vi "nanocal -- nuclear schottky fit V7.vi"() -> ()   [LabVIEW 2021] (continued)
  out "string OUT":string="  \"IDS0158_210310_RAW_cal__ref_\" ->   <|    \"ζ\" -> 0.338724462580   ,  \"τ1\" -> 0.031757745266   ,  \"τS\" -> 0.247286819047   ,  \"τN\" -> 0.322740818116   ,  \"τC\" -> 0.001034291318   ,  \"κ0\" -> 0.000000000505   ,  \"mm1\" -> 0.000261080239   ,  \"mm2\" -> 0.013473055910   ,  \"mm3\" -> 0.782167842652   ,  \"T\" -> 0.140000000000   ,  \"B\" -> 12.000000000000   ,  \"θ\" -> 0.000000000000   ,  \"Reoff\" -> -114641566.265060246000   ,  \"Imoff\" -> 0.000000000000   ,  \"στ1\" -> 0.023975320210   ,  \"στS\" -> 0.076414054009   ,  \"στN\" -> 0.076454917520    |>   , \r\"IDS0158_210310_RAW_cal__sam_\" ->   <|    \"ζ\" -> 0.286336668596   ,  \"τ1\" -> 0.037477267671   ,  \"τS\" -> 0.354459287884   ,  \"τN\" -> 0.444916383639   ,  \"τC\" -> 0.001225600579   ,  \"κ0\" -> 0.000000000596   ,  \"mm1\" -> 0.000272242393   ,  \"mm2\" -> 0.016302418461   ,  \"mm3\" -> 1.050394445660   ,  \"T\" -> 0.140000000000   ,  \"B\" -> 12.000000000000   ,  \"θ\" -> 0.000000000000   ,  \"Reoff\" -> 0.000000000000   ,  \"Imoff\" -> 0.000000000000   ,  \"στ1\" -> 0.000000000000   ,  \"στS\" -> 0.000000000000   ,  \"στN\" -> 0.000000000000    |>   , \r\"IDS0159_210310_RAW_cal__ref_\" ->   <|    \"ζ\" -> 0.271267920492   ,  \"τ1\" -> 0.029985631647   ,  \"τS\" -> 0.193691005295   ,  \"τN\" -> 0.182171075098   ,  \"τC\" -> 0.001008816819   ,  \"κ0\" -> 0.000000000648   ,  \"mm1\" -> 0.000214568285   ,  \"mm2\" -> 0.015007137955   ,  \"mm3\" -> 0.493594147559   ,  \"T\" -> 0.170000000000   ,  \"B\" -> 12.000000000000   ,  \"θ\" -> 0.000000000000   ,  \"Reoff\" -> -68518072.289156615700   ,  \"Imoff\" -> 0.000000000000   ,  \"στ1\" -> 0.012908928279   ,  \"στS\" -> 0.012278249433   ,  \"στN\" -> 0.000000000000    |>   , \r\"IDS0159_210310_RAW_cal__sam_\" ->   <|    \"ζ\" -> 0.219100303741   ,  \"τ1\" -> 0.028643012604   ,  \"τS\" -> 0.279362928811   ,  \"τN\" -> 0.246156444058   ,  \"τC\" -> 0.001272401549   ,  \"κ0\" -> 0.000000000760   ,  \"mm1\" -> 0.000227975653   ,  \"mm2\" -> 0.014929571562   ,  \"mm3\" -> 0.655418694024   ,  \"T\" -> 0.170000000000   ,  \"B\" -> 12.000000000000   ,  \"θ\" -> 0.000000000000   ,  \"Reoff\" -> 0.000000000000   ,  \"Imoff\" -> 0.000000000000   ,  \"στ1\" -> 0.000000000000   ,  \"στS\" -> 0.000000000000   ,  \"στN\" -> 0.000000000000    |>   , \r\"IDS0160_210310_RAW_cal__ref_\" ->   <|    \"ζ\" -> 0.207139977904   ,  \"τ1\" -> 0.027467343957   ,  \"τS\" -> 0.117438673826   ,  \"τN\" -> 0.102057074143   ,  \"τC\" -> 0.000949663971   ,  \"κ0\" -> 0.000000000917   ,  \"mm1\" -> 0.000162053218   ,  \"mm2\" -> 0.014024936030   ,  \"mm3\" -> 0.279192111033   ,  \"T\" -> 0.200000000000   ,  \"B\" -> 12.000000000000   ,  \"θ\" -> 0.000000000000   ,  \"Reoff\" -> -40668674.698795177000   ,  \"Imoff\" -> 0.000000000000   ,  \"στ1\" -> 0.009618369087   ,  \"στS\" -> 0.007137384425   ,  \"στN\" -> 0.000000000000    |>   , \r\"IDS0160_210310_RAW_cal__sam_\" ->   <|    \"ζ\" -> 0.170488637524   ,  \"τ1\" -> 0.029234231120   ,  \"τS\" -> 0.149095458227   ,  \"τN\" -> 0.151792620275   ,  \"τC\" -> 0.001113424175   ,  \"κ0\" -> 0.000000001042   ,  \"mm1\" -> 0.000161291869   ,  \"mm2\" -> 0.013922632736   ,  \"mm3\" -> 0.368449807743   ,  \"T\" -> 0.200000000000   ,  \"B\" -> 12.000000000000   ,  \"θ\" -> 0.000000000000   ,  \"Reoff\" -> 0.000000000000   ,  \"Imoff\" -> 0.000000000000   ,  \"στ1\" -> 0.000000000000   ,  \"στS\" -> 0.000000000000   ,  \"στN\" -> 0.000000000000    |>   , \r\"IDS0161_210310_RAW_cal__ref_\" ->   <|    \"ζ\" -> 0.165651103495   ,  \"τ1\" -> 0.025219369633   ,  \"τS\" -> 0.095243887499   ,  \"τN\" -> 0.068405844588   ,  \"τC\" -> 0.001096621932   ,  \"κ0\" -> 0.000000001058   ,  \"mm1\" -> 0.000154524257   ,  \"mm2\" -> 0.013909362731   ,  \"mm3\" -> 0.203010595371   ,  \"T\" -> 0.220000000000   ,  \"B\" -> 12.000000000000   ,  \"θ\" -> 0.000000000000   ,  \"Reoff\" -> -26138554.216867461800   ,  \"Imoff\" -> 0.000000000000   ,  \"στ1\" -> 0.007587881902   ,  \"στS\" -> 0.004844828321   ,  \"στN\" -> 0.000000000000    |>   , \r\"IDS0161_210310_RAW_cal__sam_\" ->   <|    \"ζ\" -> 0.130531197151   ,  \"τ1\" -> 0.025704482770   ,  \"τS\" -> 0.129606657196   ,  \"τN\" -> 0.091602369165   ,  \"τC\" -> 0.001441379995   ,  \"κ0\" -> 0.000000001211   ,  \"mm1\" -> 0.000164978070   ,  \"mm2\" -> 0.014468182937   ,  \"mm3\" -> 0.262596407151   ,  \"T\" -> 0.220000000000   ,  \"B\" -> 12.000000000000   ,  \"θ\" -> 0.000000000000   ,  \"Reoff\" -> 0.000000000000   ,  \"Imoff\" -> 0.000000000000   ,  \"στ1\" -> 0.000000000000   ,  \"στS\" -> 0.000000000000   ,  \"στN\" -> 0.000000000000    |>   , \r\"IDS0162_210310_RAW_cal__ref_\" ->   <|    \"ζ\" -> 0.096222034275   ,  \"τ1\" -> 0.023686784650   ,  \"τS\" -> 0.070336744639   ,  \"τN\" -> 0.023939989572   ,  \"τC\" -> 0.001388596335   ,  \"κ0\" -> 0.000000001367   ,  \"mm1\" -> 0.000119909077   ,  \"mm2\" -> 0.016622969082   ,  \"mm3\" -> 0.111680736187   ,  \"T\" -> 0.280000000000   ,  \"B\" -> 12.000000000000   ,  \"θ\" -> 0.000000000000   ,  \"Reoff\" -> -11003012.048192769300   ,  \"Imoff\" -> 0.000000000000   ,  \"στ1\" -> 0.008753356754   ,  \"στS\" -> 0.002669913437   ,  \"στN\" -> 0.000000000000    |>   , \r\"IDS0162_210310_RAW_cal__sam_\" ->   <|    \"ζ\" -> 0.078258046754   ,  \"τ1\" -> 0.028009840731   ,  \"τS\" -> 0.092122038762   ,  \"τN\" -> 0.030129595899   ,  \"τC\" -> 0.001641062244   ,  \"κ0\" -> 0.000000001543   ,  \"mm1\" -> 0.000117303440   ,  \"mm2\" -> 0.019983073008   ,  \"mm3\" -> 0.141369335330   ,  \"T\" -> 0.280000000000   ,  \"B\" -> 12.000000000000   ,  \"θ\" -> 0.000000000000   ,  \"Reoff\" -> 0.000000000000   ,  \"Imoff\" -> 0.000000000000   ,  \"στ1\" -> 0.000000000000   ,  \"στS\" -> 0.000000000000   ,  \"στN\" -> 0.000000000000    |>   , \r\"IDS0163_210310_RAW_cal__ref_\" ->   <|    \"ζ\" -> 0.066672200447   ,  \"τ1\" -> 0.021639337174   ,  \"τS\" -> 0.054330230678   ,  \"τN\" -> 0.012190158529   ,  \"τC\" -> 0.001673698086   ,  \"κ0\" -> 0.000000001744   ,  \"mm1\" -> 0.000101848885   ,  \"mm2\" -> 0.016608176692   ,  \"mm3\" -> 0.077558459612   ,  \"T\" -> 0.330000000000   ,  \"B\" -> 12.000000000000   ,  \"θ\" -> 0.000000000000   ,  \"Reoff\" -> -6192771.084337353710   ,  \"Imoff\" -> 0.000000000000   ,  \"στ1\" -> 0.010795838687   ,  \"στS\" -> 0.002003612837   ,  \"στN\" -> 0.000000000000    |>   , \r\"IDS0163_210310_RAW_cal__sam_\" ->   <|    \"ζ\" -> 0.054088186012   ,  \"τ1\" -> 0.023838802615   ,  \"τS\" -> 0.069079396629   ,  \"τN\" -> 0.016435267456   ,  \"τC\" -> 0.002025071743   ,  \"κ0\" -> 0.000000001955   ,  \"mm1\" -> 0.000101234646   ,  \"mm2\" -> 0.018244822177   ,  \"mm3\" -> 0.097657814678   ,  \"T\" -> 0.330000000000   ,  \"B\" -> 12.000000000000   ,  \"θ\" -> 0.000000000000   ,  \"Reoff\" -> 0.000000000000   ,  \"Imoff\" -> 0.000000000000   ,  \"στ1\" -> 0.000000000000   ,  \"στS\" -> 0.000000000000   ,  \"στN\" -> 0.000000000000    |>   , \r\"IDS0164_210310_RAW_cal__ref_\" ->   <|    \"ζ\" -> 0.047185670549   ,  \"τ1\" -> 0.020999787986   ,  \"τS\" -> 0.044123234525   ,  \"τN\" -> 0.006414229914   ,  \"τC\" -> 0.002330922094   ,  \"κ0\" -> 0.000000002161   ,  \"mm1\" -> 0.000100189786   ,  \"mm2\" -> 0.017276594586   ,  \"mm3\" -> 0.058876034294   ,  \"T\" -> 0.400000000000   ,  \"B\" -> 12.000000000000   ,  \"θ\" -> 0.000000000000   ,  \"Reoff\" -> -3126506.024096369740   ,  \"Imoff\" -> 0.000000000000   ,  \"στ1\" -> 0.014319461595   ,  \"στS\" -> 0.001588428387   ,  \"στN\" -> 0.000000000000    |>   , \r\"IDS0164_210310_RAW_cal__sam_\" ->   <|    \"ζ\" -> 0.039314966212   ,  \"τ1\" -> 0.020712803909   ,  \"τS\" -> 0.055413767550   ,  \"τN\" -> 0.008474403424   ,  \"τC\" -> 0.002674063387   ,  \"κ0\" -> 0.000000002415   ,  \"mm1\" -> 0.000096818147   ,  \"mm2\" -> 0.017190811405   ,  \"mm3\" -> 0.072499170001   ,  \"T\" -> 0.400000000000   ,  \"B\" -> 12.000000000000   ,  \"θ\" -> 0.000000000000   ,  \"Reoff\" -> 0.000000000000   ,  \"Imoff\" -> 0.000000000000   ,  \"στ1\" -> 0.000000000000   ,  \"στS\" -> 0.000000000000   ,  \"στN\" -> 0.000000000000    |>   , \r\"IDS0165_210310_RAW_cal__ref_\" ->   <|    \"ζ\" -> 0.033577393126   ,  \"τ1\" -> 0.018946820322   ,  \"τS\" -> 0.035749921348   ,  \"τN\" -> 0.004008447047   ,  \"τC\" -> 0.003122429757   ,  \"κ0\" -> 0.000000002680   ,  \"mm1\" -> 0.000093748549   ,  \"mm2\" -> 0.016142439680   ,  \"mm3\" -> 0.046926412611   ,  \"T\" -> 0.480000000000   ,  \"B\" -> 12.000000000000   ,  \"θ\" -> 0.000000000000   ,  \"Reoff\" -> -1313253.012048184870   ,  \"Imoff\" -> 0.000000000000   ,  \"στ1\" -> 0.017565086331   ,  \"στS\" -> 0.001375721175   ,  \"στN\" -> 0.000000000000    |>   , \r\"IDS0165_210310_RAW_cal__sam_\" ->   <|    \"ζ\" -> 0.031945976845   ,  \"τ1\" -> 0.019000922826   ,  \"τS\" -> 0.045624146388   ,  \"τN\" -> 0.005314716063   ,  \"τC\" -> 0.002488383471   ,  \"κ0\" -> 0.000000002954   ,  \"mm1\" -> 0.000073272643   ,  \"mm2\" -> 0.016306894362   ,  \"mm3\" -> 0.057675293464   ,  \"T\" -> 0.480000000000   ,  \"B\" -> 12.000000000000   ,  \"θ\" -> 0.000000000000   ,  \"Reoff\" -> 0.000000000000   ,  \"Imoff\" -> 0.000000000000   ,  \"στ1\" -> 0.000000000000   ,  \"στS\" -> 0.000000000000   ,  \"στN\" -> 0.000000000000    |>   , \r\"IDS0166_210310_RAW_cal__ref_\" ->   <|    \"ζ\" -> 0.026134408941   ,  \"τ1\" -> 0.018837221506   ,  \"τS\" -> 0.029046436266   ,  \"τN\" -> 0.002475934064   ,  \"τC\" -> 0.003637611641   ,  \"κ0\" -> 0.000000003369   ,  \"mm1\" -> 0.000082770074   ,  \"mm2\" -> 0.016386102123   ,  \"mm3\" -> 0.038352149797   ,  \"T\" -> 0.580000000000   ,  \"B\" -> 12.000000000000   ,  \"θ\" -> 0.000000000000   ,  \"Reoff\" -> -406626.506024092435   ,  \"Imoff\" -> 0.000000000000   ,  \"στ1\" -> 0.034768871814   ,  \"στS\" -> 0.001627850434   ,  \"στN\" -> 0.000000000000    |>   , \r\"IDS0166_210310_RAW_cal__sam_\" ->   <|    \"ζ\" -> 0.023031239946   ,  \"τ1\" -> 0.018268814012   ,  \"τS\" -> 0.037269400776   ,  \"τN\" -> 0.002696792890   ,  \"τC\" -> 0.003257395394   ,  \"κ0\" -> 0.000000003720   ,  \"mm1\" -> 0.000067670174   ,  \"mm2\" -> 0.016445281937   ,  \"mm3\" -> 0.045899921957   ,  \"T\" -> 0.580000000000   ,  \"B\" -> 12.000000000000   ,  \"θ\" -> 0.000000000000   ,  \"Reoff\" -> 0.000000000000   ,  \"Imoff\" -> 0.000000000000   ,  \"στ1\" -> 0.000000000000   ,  \"στS\" -> 0.000000000000   ,  \"στN\" -> 0.000000000000    |>   , \r\"IDS0167_210310_RAW_cal__ref_\" ->   <|    \"ζ\" -> 0.026557278794   ,  \"τ1\" -> 0.016933945977   ,  \"τS\" -> 0.022881111855   ,  \"τN\" -> 0.001392473895   ,  \"τC\" -> 0.004119437148   ,  \"κ0\" -> 0.000000003981   ,  \"mm1\" -> 0.000090964667   ,  \"mm2\" -> 0.015177563241   ,  \"mm3\" -> 0.030703081351   ,  \"T\" -> 0.680000000000   ,  \"B\" -> 12.000000000000   ,  \"θ\" -> 0.000000000000   ,  \"Reoff\" -> 0.000000000000   ,  \"Imoff\" -> 0.000000000000   ,  \"στ1\" -> 0.000000000000   ,  \"στS\" -> 0.000000000000   ,  \"στN\" -> 0.000000000000    |>   , \r\"IDS0167_210310_RAW_cal__sam_\" ->   <|    \"ζ\" -> 0.019920170845   ,  \"τ1\" -> 0.016368892412   ,  \"τS\" -> 0.030579536580   ,  \"τN\" -> 0.001736017565   ,  \"τC\" -> 0.004971418152   ,  \"κ0\" -> 0.000000004410   ,  \"mm1\" -> 0.000083939556   ,  \"mm2\" -> 0.015095997595   ,  \"mm3\" -> 0.039119658918   ,  \"T\" -> 0.680000000000   ,  \"B\" -> 12.000000000000   ,  \"θ\" -> 0.000000000000   ,  \"Reoff\" -> 0.000000000000   ,  \"Imoff\" -> 0.000000000000   ,  \"στ1\" -> 0.000000000000   ,  \"στS\" -> 0.000000000000   ,  \"στN\" -> 0.000000000000    |>   , \r\"IDS0168_210310_RAW_cal__ref_\" ->   <|    \"ζ\" -> 0.022041296958   ,  \"τ1\" -> 0.014045615335   ,  \"τS\" -> 0.018889590451   ,  \"τN\" -> 0.000813465770   ,  \"τC\" -> 0.004122617309   ,  \"κ0\" -> 0.000000005540   ,  \"mm1\" -> 0.000073491061   ,  \"mm2\" -> 0.013002629707   ,  \"mm3\" -> 0.025229449010   ,  \"T\" -> 0.910000000000   ,  \"B\" -> 12.000000000000   ,  \"θ\" -> 0.000000000000   ,  \"Reoff\" -> 0.000000000000   ,  \"Imoff\" -> 0.000000000000   ,  \"στ1\" -> 0.000000000000   ,  \"στS\" -> 0.000000000000   ,  \"στN\" -> 0.000000000000    |>   , \r\"IDS0168_210310_RAW_cal__sam_\" ->   <|    \"ζ\" -> 0.017558473054   ,  \"τ1\" -> 0.014545104284   ,  \"τS\" -> 0.022979681288   ,  \"τN\" -> 0.000840829385   ,  \"τC\" -> 0.005228030240   ,  \"κ0\" -> 0.000000006068   ,  \"mm1\" -> 0.000073916527   ,  \"mm2\" -> 0.013750428362   ,  \"mm3\" -> 0.030187552103   ,  \"T\" -> 0.910000000000   ,  \"B\" -> 12.000000000000   ,  \"θ\" -> 0.000000000000   ,  \"Reoff\" -> 0.000000000000   ,  \"Imoff\" -> 0.000000000000   ,  \"στ1\" -> 0.000000000000   ,  \"στS\" -> 0.000000000000   ,  \"στN\" -> 0.000000000000    |>   , \r\"IDS0169_210310_RAW_cal__ref_\" ->   <|    \"ζ\" -> 0.021090283514   ,  \"τ1\" -> 0.013945744068   ,  \"τS\" -> 0.014386606899   ,  \"τN\" -> 0.000345175874   ,  \"τC\" -> 0.004902956629   ,  \"κ0\" -> 0.000000007742   ,  \"mm1\" -> 0.000076221408   ,  \"mm2\" -> 0.013209066715   ,  \"mm3\" -> 0.020605892822   ,  \"T\" -> 1.230000000000   ,  \"B\" -> 12.000000000000   ,  \"θ\" -> 0.000000000000   ,  \"Reoff\" -> 0.000000000000   ,  \"Imoff\" -> 0.000000000000   ,  \"στ1\" -> 0.000000000000   ,  \"στS\" -> 0.000000000000   ,  \"στN\" -> 0.000000000000    |>   , \r\"IDS0169_210310_RAW_cal__sam_\" ->   <|    \"ζ\" -> 0.011916480594   ,  \"τ1\" -> 0.012551282481   ,  \"τS\" -> 0.018233218660   ,  \"τN\" -> 0.000345702746   ,  \"τC\" -> 0.004699451527   ,  \"κ0\" -> 0.000000008451   ,  \"mm1\" -> 0.000044190864   ,  \"mm2\" -> 0.012162820727   ,  \"mm3\" -> 0.023844039179   ,  \"T\" -> 1.230000000000   ,  \"B\" -> 12.000000000000   ,  \"θ\" -> 0.000000000000   ,  \"Reoff\" -> 0.000000000000   ,  \"Imoff\" -> 0.000000000000   ,  \"στ1\" -> 0.000000000000   ,  \"στS\" -> 0.000000000000   ,  \"στN\" -> 0.000000000000    |>   , \r\"IDS0170_210310_RAW_cal__ref_\" ->   <|    \"ζ\" -> 0.021449250230   ,  \"τ1\" -> 0.014564522147   ,  \"τS\" -> 0.008878867204   ,  \"τN\" -> 0.000064984242   ,  \"τC\" -> 0.006207353748   ,  \"κ0\" -> 0.000000012530   ,  \"mm1\" -> 0.000077778127   ,  \"mm2\" -> 0.013872772336   ,  \"mm3\" -> 0.015957015786   ,  \"T\" -> 1.970000000000   ,  \"B\" -> 12.000000000000   ,  \"θ\" -> 0.000000000000   ,  \"Reoff\" -> 0.000000000000   ,  \"Imoff\" -> 0.000000000000   ,  \"στ1\" -> 0.000000000000   ,  \"στS\" -> 0.000000000000   ,  \"στN\" -> 0.000000000000    |>   , \r\"IDS0170_210310_RAW_cal__sam_\" ->   <|    \"ζ\" -> 0.012831327568   ,  \"τ1\" -> 0.013315909415   ,  \"τS\" -> 0.012590836847   ,  \"τN\" -> 0.000065003013   ,  \"τC\" -> 0.005276356243   ,  \"κ0\" -> 0.000000013610   ,  \"mm1\" -> 0.000047406274   ,  \"mm2\" -> 0.013137605540   ,  \"mm3\" -> 0.018225484932   ,  \"T\" -> 1.970000000000   ,  \"B\" -> 12.000000000000   ,  \"θ\" -> 0.000000000000   ,  \"Reoff\" -> 0.000000000000   ,  \"Imoff\" -> 0.000000000000   ,  \"στ1\" -> 0.000000000000   ,  \"στS\" -> 0.000000000000   ,  \"στN\" -> 0.000000000000    |>   , \r\"IDS0171_210310_RAW_cal__ref_\" ->   <|    \"ζ\" -> 0.024633693577   ,  \"τ1\" -> 0.014940694735   ,  \"τS\" -> 0.006137734482   ,  \"τN\" -> 0.000014567254   ,  \"τC\" -> 0.005080683927   ,  \"κ0\" -> 0.000000022488   ,  \"mm1\" -> 0.000067969819   ,  \"mm2\" -> 0.011256263587   ,  \"mm3\" -> 0.015001000908   ,  \"T\" -> 3.190000000000   ,  \"B\" -> 12.000000000000   ,  \"θ\" -> 0.000000000000   ,  \"Reoff\" -> 0.000000000000   ,  \"Imoff\" -> 0.000000000000   ,  \"στ1\" -> 0.000000000000   ,  \"στS\" -> 0.000000000000   ,  \"στN\" -> 0.000000000000    |>   , \r\"IDS0171_210310_RAW_cal__sam_\" ->   <|    \"ζ\" -> 0.019774146838   ,  \"τ1\" -> 0.013257273421   ,  \"τS\" -> 0.007064131508   ,  \"τN\" -> 0.000028000819   ,  \"τC\" -> 0.006942241845   ,  \"κ0\" -> 0.000000023477   ,  \"mm1\" -> 0.000068886863   ,  \"mm2\" -> 0.012935419574   ,  \"mm3\" -> 0.014427582022   ,  \"T\" -> 3.190000000000   ,  \"B\" -> 12.000000000000   ,  \"θ\" -> 0.000000000000   ,  \"Reoff\" -> 0.000000000000   ,  \"Imoff\" -> 0.000000000000   ,  \"στ1\" -> 0.000000000000   ,  \"στS\" -> 0.000000000000   ,  \"στN\" -> 0.000000000000    |>   , \r\"IDS0172_210310_RAW_cal__ref_\" ->   <|    \"ζ\" -> 0.027835388666   ,  \"τ1\" -> 0.013976390421   ,  \"τS\" -> 0.003539188638   ,  \"τN\" -> 0.000003774856   ,  \"τC\" -> 0.004420299329   ,  \"κ0\" -> 0.000000055482   ,  \"mm1\" -> 0.000054408485   ,  \"mm2\" -> 0.007998445403   ,  \"mm3\" -> 0.013985419121   ,  \"T\" -> 5.800000000000   ,  \"B\" -> 12.000000000000   ,  \"θ\" -> 0.000000000000   ,  \"Reoff\" -> 0.000000000000   ,  \"Imoff\" -> 0.000000000000   ,  \"στ1\" -> 0.000000000000   ,  \"στS\" -> 0.000000000000   ,  \"στN\" -> 0.000000000000    |>   , \r\"IDS0172_210310_RAW_cal__sam_\" ->   <|    \"ζ\" -> 0.029251354442   ,  \"τ1\" -> 0.014634751206   ,  \"τS\" -> 0.003873958746   ,  \"τN\" -> 0.000007000487   ,  \"τC\" -> 0.006827504775   ,  \"κ0\" -> 0.000000056438   ,  \"mm1\" -> 0.000072018576   ,  \"mm2\" -> 0.010723236476   ,  \"mm3\" -> 0.014661483476   ,  \"T\" -> 5.800000000000   ,  \"B\" -> 12.000000000000   ,  \"θ\" -> 0.000000000000   ,  \"Reoff\" -> 0.000000000000   ,  \"Imoff\" -> 0.000000000000   ,  \"στ1\" -> 0.000000000000   ,  \"στS\" -> 0.000000000000   ,  \"στN\" -> 0.000000000000    |>   , \r\"IDS0181_210310_RAW_cal__ref_\" ->   <|    \"ζ\" -> 0.196256884521   ,  \"τ1\" -> 0.071380539398   ,  \"τS\" -> 0.034448108903   ,  \"τN\" -> 0.119444210569   ,  \"τC\" -> 0.001245873609   ,  \"κ0\" -> 0.000000000908   ,  \"mm1\" -> 0.000199286041   ,  \"mm2\" -> 0.012356130491   ,  \"mm3\" -> 0.244165743118   ,  \"T\" -> 0.179000000000   ,  \"B\" -> 12.000000000000   ,  \"θ\" -> 90.000000000000   ,  \"Reoff\" -> -32111445.783132523300   ,  \"Imoff\" -> 0.000000000000   ,  \"στ1\" -> 0.005873597921   ,  \"στS\" -> 0.002285203630   ,  \"στN\" -> 0.000000000000    |>   , \r\"IDS0181_210310_RAW_cal__sam_\" ->   <|    \"ζ\" -> 0.161975781729   ,  \"τ1\" -> 0.073089805113   ,  \"τS\" -> 0.045018408115   ,  \"τN\" -> 0.161987434028   ,  \"τC\" -> 0.001482104484   ,  \"κ0\" -> 0.000000001038   ,  \"mm1\" -> 0.000201615809   ,  \"mm2\" -> 0.012976126678   ,  \"mm3\" -> 0.301929942357   ,  \"T\" -> 0.179000000000   ,  \"B\" -> 12.000000000000   ,  \"θ\" -> 90.000000000000   ,  \"Reoff\" -> 0.000000000000   ,  \"Imoff\" -> 0.000000000000   ,  \"στ1\" -> 0.000000000000   ,  \"στS\" -> 0.000000000000   ,  \"στN\" -> 0.000000000000    |>   , \r\"IDS0183_210310_RAW_cal__ref_\" ->   <|    \"ζ\" -> 0.374777480634   ,  \"τ1\" -> 0.116873786162   ,  \"τS\" -> 0.055337513541   ,  \"τN\" -> 0.665911779860   ,  \"τC\" -> 0.001012065497   ,  \"κ0\" -> 0.000000000453   ,  \"mm1\" -> 0.000273168605   ,  \"mm2\" -> 0.008156341144   ,  \"mm3\" -> 1.101013628401   ,  \"T\" -> 0.120000000000   ,  \"B\" -> 12.000000000000   ,  \"θ\" -> 90.000000000000   ,  \"Reoff\" -> -135984939.759036154000   ,  \"Imoff\" -> 0.000000000000   ,  \"στ1\" -> 0.014306498614   ,  \"στS\" -> 0.016176400349   ,  \"στN\" -> 0.000000000000    |>   , \r\"IDS0183_210310_RAW_cal__sam_\" ->   <|    \"ζ\" -> 0.300863384227   ,  \"τ1\" -> 0.104924004009   ,  \"τS\" -> 0.071070599729   ,  \"τN\" -> 0.992887187112   ,  \"τC\" -> 0.001721587800   ,  \"κ0\" -> 0.000000000548   ,  \"mm1\" -> 0.000392216822   ,  \"mm2\" -> 0.006637384427   ,  \"mm3\" -> 1.483679717825   ,  \"T\" -> 0.120000000000   ,  \"B\" -> 12.000000000000   ,  \"θ\" -> 90.000000000000   ,  \"Reoff\" -> 0.000000000000   ,  \"Imoff\" -> 0.000000000000   ,  \"στ1\" -> 0.000000000000   ,  \"στS\" -> 0.000000000000   ,  \"στN\" -> 0.000000000000    |>   , \r\"IDS0184_210310_RAW_cal__ref_\" ->   <|    \"ζ\" -> 0.262136034943   ,  \"τ1\" -> 0.088367137171   ,  \"τS\" -> 0.043836416470   ,  \"τN\" -> 0.254908544273   ,  \"τC\" -> 0.001163145607   ,  \"κ0\" -> 0.000000000664   ,  \"mm1\" -> 0.000237539268   ,  \"mm2\" -> 0.010917614909   ,  \"mm3\" -> 0.455431908812   ,  \"T\" -> 0.148000000000   ,  \"B\" -> 12.000000000000   ,  \"θ\" -> 90.000000000000   ,  \"Reoff\" -> -57475903.614457845700   ,  \"Imoff\" -> 0.000000000000   ,  \"στ1\" -> 0.008732968552   ,  \"στS\" -> 0.004342493905   ,  \"στN\" -> 0.000000000000    |>   , \r\"IDS0184_210310_RAW_cal__sam_\" ->   <|    \"ζ\" -> 0.215697702358   ,  \"τ1\" -> 0.095971807771   ,  \"τS\" -> 0.069319630290   ,  \"τN\" -> 0.366712218878   ,  \"τC\" -> 0.001526252261   ,  \"κ0\" -> 0.000000000784   ,  \"mm1\" -> 0.000266752031   ,  \"mm2\" -> 0.013373263674   ,  \"mm3\" -> 0.613940961515   ,  \"T\" -> 0.148000000000   ,  \"B\" -> 12.000000000000   ,  \"θ\" -> 90.000000000000   ,  \"Reoff\" -> 0.000000000000   ,  \"Imoff\" -> 0.000000000000   ,  \"στ1\" -> 0.000000000000   ,  \"στS\" -> 0.000000000000   ,  \"στN\" -> 0.000000000000    |>   , \r\"IDS0185_210310_RAW_cal__ref_\" ->   <|    \"ζ\" -> 0.167787986703   ,  \"τ1\" -> 0.066347554389   ,  \"τS\" -> 0.031904428619   ,  \"τN\" -> 0.087950028761   ,  \"τC\" -> 0.001302549579   ,  \"κ0\" -> 0.000000001074   ,  \"mm1\" -> 0.000181644072   ,  \"mm2\" -> 0.013106205618   ,  \"mm3\" -> 0.194326849759   ,  \"T\" -> 0.197000000000   ,  \"B\" -> 12.000000000000   ,  \"θ\" -> 90.000000000000   ,  \"Reoff\" -> -23656626.506024092400   ,  \"Imoff\" -> 0.000000000000   ,  \"στ1\" -> 0.005345315984   ,  \"στS\" -> 0.001758488229   ,  \"στN\" -> 0.000000000000    |>   , \r\"IDS0185_210310_RAW_cal__sam_\" ->   <|    \"ζ\" -> 0.139117463690   ,  \"τ1\" -> 0.070330410174   ,  \"τS\" -> 0.040829719954   ,  \"τN\" -> 0.122434321115   ,  \"τC\" -> 0.001436112939   ,  \"κ0\" -> 0.000000001208   ,  \"mm1\" -> 0.000170710071   ,  \"mm2\" -> 0.013785404893   ,  \"mm3\" -> 0.243787328523   ,  \"T\" -> 0.197000000000   ,  \"B\" -> 12.000000000000   ,  \"θ\" -> 90.000000000000   ,  \"Reoff\" -> 0.000000000000   ,  \"Imoff\" -> 0.000000000000   ,  \"στ1\" -> 0.000000000000   ,  \"στS\" -> 0.000000000000   ,  \"στN\" -> 0.000000000000    |>   , \r\"IDS0186_210310_RAW_cal__ref_\" ->   <|    \"ζ\" -> 0.101010290290   ,  \"τ1\" -> 0.051600602883   ,  \"τS\" -> 0.026928622174   ,  \"τN\" -> 0.035515045222   ,  \"τC\" -> 0.001497230367   ,  \"κ0\" -> 0.000000001365   ,  \"mm1\" -> 0.000131291688   ,  \"mm2\" -> 0.014998326833   ,  \"mm3\" -> 0.106719335096   ,  \"T\" -> 0.249000000000   ,  \"B\" -> 12.000000000000   ,  \"θ\" -> 90.000000000000   ,  \"Reoff\" -> -12786144.578313261300   ,  \"Imoff\" -> 0.000000000000   ,  \"στ1\" -> 0.005301578025   ,  \"στS\" -> 0.001106289912   ,  \"στN\" -> 0.000000000000    |>   , \r\"IDS0186_210310_RAW_cal__sam_\" ->   <|    \"ζ\" -> 0.079912790251   ,  \"τ1\" -> 0.053932962768   ,  \"τS\" -> 0.033847624645   ,  \"τN\" -> 0.047947649984   ,  \"τC\" -> 0.001828917906   ,  \"κ0\" -> 0.000000001546   ,  \"mm1\" -> 0.000129305669   ,  \"mm2\" -> 0.016142481427   ,  \"mm3\" -> 0.127821856832   ,  \"T\" -> 0.249000000000   ,  \"B\" -> 12.000000000000   ,  \"θ\" -> 90.000000000000   ,  \"Reoff\" -> 0.000000000000   ,  \"Imoff\" -> 0.000000000000   ,  \"στ1\" -> 0.000000000000   ,  \"στS\" -> 0.000000000000   ,  \"στN\" -> 0.000000000000    |>   , \r\"IDS0187_210310_RAW_cal__ref_\" ->   <|    \"ζ\" -> 0.070400852728   ,  \"τ1\" -> 0.043683571138   ,  \"τS\" -> 0.023747872987   ,  \"τN\" -> 0.017566907569   ,  \"τC\" -> 0.001811397979   ,  \"κ0\" -> 0.000000001742   ,  \"mm1\" -> 0.000111656339   ,  \"mm2\" -> 0.016123687864   ,  \"mm3\" -> 0.073483001252   ,  \"T\" -> 0.300000000000   ,  \"B\" -> 12.000000000000   ,  \"θ\" -> 90.000000000000   ,  \"Reoff\" -> -7469879.518072288490   ,  \"Imoff\" -> 0.000000000000   ,  \"στ1\" -> 0.006425128340   ,  \"στS\" -> 0.000860913040   ,  \"στN\" -> 0.000000000000    |>   , \r\"IDS0187_210310_RAW_cal__sam_\" ->   <|    \"ζ\" -> 0.057938569833   ,  \"τ1\" -> 0.045244527663   ,  \"τS\" -> 0.029709028064   ,  \"τN\" -> 0.023577376257   ,  \"τC\" -> 0.002006607539   ,  \"κ0\" -> 0.000000001948   ,  \"mm1\" -> 0.000103608352   ,  \"mm2\" -> 0.017542867394   ,  \"mm3\" -> 0.085978401835   ,  \"T\" -> 0.300000000000   ,  \"B\" -> 12.000000000000   ,  \"θ\" -> 90.000000000000   ,  \"Reoff\" -> 0.000000000000   ,  \"Imoff\" -> 0.000000000000   ,  \"στ1\" -> 0.000000000000   ,  \"στS\" -> 0.000000000000   ,  \"στN\" -> 0.000000000000    |>   , \r\"IDS0188_210310_RAW_cal__ref_\" ->   <|    \"ζ\" -> 0.052056900695   ,  \"τ1\" -> 0.037832738296   ,  \"τS\" -> 0.021653292165   ,  \"τN\" -> 0.010363134799   ,  \"τC\" -> 0.002302160053   ,  \"κ0\" -> 0.000000002117   ,  \"mm1\" -> 0.000103876216   ,  \"mm2\" -> 0.016526845939   ,  \"mm3\" -> 0.057187279117   ,  \"T\" -> 0.360000000000   ,  \"B\" -> 12.000000000000   ,  \"θ\" -> 90.000000000000   ,  \"Reoff\" -> -4033132.530120491980   ,  \"Imoff\" -> 0.000000000000   ,  \"στ1\" -> 0.008023460591   ,  \"στS\" -> 0.000770743330   ,  \"στN\" -> 0.000000000000    |>   , \r\"IDS0188_210310_RAW_cal__sam_\" ->   <|    \"ζ\" -> 0.044154556051   ,  \"τ1\" -> 0.038823125235   ,  \"τS\" -> 0.027069314930   ,  \"τN\" -> 0.013601990730   ,  \"τC\" -> 0.002287979276   ,  \"κ0\" -> 0.000000002359   ,  \"mm1\" -> 0.000089763345   ,  \"mm2\" -> 0.018083678254   ,  \"mm3\" -> 0.065404792018   ,  \"T\" -> 0.360000000000   ,  \"B\" -> 12.000000000000   ,  \"θ\" -> 90.000000000000   ,  \"Reoff\" -> 0.000000000000   ,  \"Imoff\" -> 0.000000000000   ,  \"στ1\" -> 0.000000000000   ,  \"στS\" -> 0.000000000000   ,  \"στN\" -> 0.000000000000    |>   , \r\"IDS0189_210310_RAW_cal__ref_\" ->   <|    \"ζ\" -> 0.040604780260   ,  \"τ1\" -> 0.030361089686   ,  \"τS\" -> 0.019771781814   ,  \"τN\" -> 0.005325171714   ,  \"τC\" -> 0.002699153711   ,  \"κ0\" -> 0.000000002668   ,  \"mm1\" -> 0.000093474055   ,  \"mm2\" -> 0.016547199805   ,  \"mm3\" -> 0.042535579348   ,  \"T\" -> 0.430000000000   ,  \"B\" -> 12.000000000000   ,  \"θ\" -> 90.000000000000   ,  \"Reoff\" -> -3126506.024096369740   ,  \"Imoff\" -> 0.000000000000   ,  \"στ1\" -> 0.010974863923   ,  \"στS\" -> 0.000726728157   ,  \"στN\" -> 0.000000000000    |>   , \r\"IDS0189_210310_RAW_cal__sam_\" ->   <|    \"ζ\" -> 0.032748569996   ,  \"τ1\" -> 0.031072007290   ,  \"τS\" -> 0.024343937548   ,  \"τN\" -> 0.006961654481   ,  \"τC\" -> 0.002967111565   ,  \"κ0\" -> 0.000000002964   ,  \"mm1\" -> 0.000084402249   ,  \"mm2\" -> 0.018055855929   ,  \"mm3\" -> 0.048229666078   ,  \"T\" -> 0.430000000000   ,  \"B\" -> 12.000000000000   ,  \"θ\" -> 90.000000000000   ,  \"Reoff\" -> 0.000000000000   ,  \"Imoff\" -> 0.000000000000   ,  \"στ1\" -> 0.000000000000   ,  \"στS\" -> 0.000000000000   ,  \"στN\" -> 0.000000000000    |>   , \r\"IDS0190_210310_RAW_cal__ref_\" ->   <|    \"ζ\" -> 0.030700897923   ,  \"τ1\" -> 0.026935085078   ,  \"τS\" -> 0.018364864329   ,  \"τN\" -> 0.002898516959   ,  \"τC\" -> 0.003150649099   ,  \"κ0\" -> 0.000000003342   ,  \"mm1\" -> 0.000080744936   ,  \"mm2\" -> 0.016939553323   ,  \"mm3\" -> 0.034981622105   ,  \"T\" -> 0.512000000000   ,  \"B\" -> 12.000000000000   ,  \"θ\" -> 90.000000000000   ,  \"Reoff\" -> 0.000000000000   ,  \"Imoff\" -> 0.000000000000   ,  \"στ1\" -> 0.000000000000   ,  \"στS\" -> 0.000000000000   ,  \"στN\" -> 0.000000000000    |>   , \r\"IDS0190_210310_RAW_cal__sam_\" ->   <|    \"ζ\" -> 0.027599263457   ,  \"τ1\" -> 0.026239105728   ,  \"τS\" -> 0.022370859308   ,  \"τN\" -> 0.003857632966   ,  \"τC\" -> 0.003499360499   ,  \"κ0\" -> 0.000000003681   ,  \"mm1\" -> 0.000081816106   ,  \"mm2\" -> 0.017901054668   ,  \"mm3\" -> 0.038707974796   ,  \"T\" -> 0.512000000000   ,  \"B\" -> 12.000000000000   ,  \"θ\" -> 90.000000000000   ,  \"Reoff\" -> 0.000000000000   ,  \"Imoff\" -> 0.000000000000   ,  \"στ1\" -> 0.000000000000   ,  \"στS\" -> 0.000000000000   ,  \"στN\" -> 0.000000000000    |>   , \r\"IDS0191_210310_RAW_cal__ref_\" ->   <|    \"ζ\" -> 0.025322625458   ,  \"τ1\" -> 0.023401812401   ,  \"τS\" -> 0.017347416709   ,  \"τN\" -> 0.002020498851   ,  \"τC\" -> 0.003594259467   ,  \"κ0\" -> 0.000000003970   ,  \"mm1\" -> 0.000074098080   ,  \"mm2\" -> 0.016429541452   ,  \"mm3\" -> 0.030350794367   ,  \"T\" -> 0.610000000000   ,  \"B\" -> 12.000000000000   ,  \"θ\" -> 90.000000000000   ,  \"Reoff\" -> 0.000000000000   ,  \"Imoff\" -> 0.000000000000   ,  \"στ1\" -> 0.000000000000   ,  \"στS\" -> 0.000000000000   ,  \"στN\" -> 0.000000000000    |>   , \r\"IDS0191_210310_RAW_cal__sam_\" ->   <|    \"ζ\" -> 0.020568815513   ,  \"τ1\" -> 0.023045965648   ,  \"τS\" -> 0.020791387386   ,  \"τN\" -> 0.002229171297   ,  \"τC\" -> 0.004427475438   ,  \"κ0\" -> 0.000000004398   ,  \"mm1\" -> 0.000074037290   ,  \"mm2\" -> 0.017820522459   ,  \"mm3\" -> 0.033072945644   ,  \"T\" -> 0.610000000000   ,  \"B\" -> 12.000000000000   ,  \"θ\" -> 90.000000000000   ,  \"Reoff\" -> 0.000000000000   ,  \"Imoff\" -> 0.000000000000   ,  \"στ1\" -> 0.000000000000   ,  \"στS\" -> 0.000000000000   ,  \"στN\" -> 0.000000000000    |>   , \r\"IDS0192_210310_RAW_cal__ref_\" ->   <|    \"ζ\" -> 0.022100596026   ,  \"τ1\" -> 0.020519097823   ,  \"τS\" -> 0.015555141042   ,  \"τN\" -> 0.000889956832   ,  \"τC\" -> 0.004354791503   ,  \"κ0\" -> 0.000000005560   ,  \"mm1\" -> 0.000074184851   ,  \"mm2\" -> 0.016476573734   ,  \"mm3\" -> 0.025131675080   ,  \"T\" -> 0.810000000000   ,  \"B\" -> 12.000000000000   ,  \"θ\" -> 90.000000000000   ,  \"Reoff\" -> 0.000000000000   ,  \"Imoff\" -> 0.000000000000   ,  \"στ1\" -> 0.000000000000   ,  \"στS\" -> 0.000000000000   ,  \"στN\" -> 0.000000000000    |>   , \r\"IDS0192_210310_RAW_cal__sam_\" ->   <|    \"ζ\" -> 0.016548170999   ,  \"τ1\" -> 0.020108887890   ,  \"τS\" -> 0.018558394948   ,  \"τN\" -> 0.001160732495   ,  \"τC\" -> 0.004746126241   ,  \"κ0\" -> 0.000000005882   ,  \"mm1\" -> 0.000061890920   ,  \"mm2\" -> 0.017029753868   ,  \"mm3\" -> 0.027808812278   ,  \"T\" -> 0.810000000000   ,  \"B\" -> 12.000000000000   ,  \"θ\" -> 90.000000000000   ,  \"Reoff\" -> 0.000000000000   ,  \"Imoff\" -> 0.000000000000   ,  \"στ1\" -> 0.000000000000   ,  \"στS\" -> 0.000000000000   ,  \"στN\" -> 0.000000000000    |>   , \r\"IDS0193_210310_RAW_cal__ref_\" ->   <|    \"ζ\" -> 0.020969814378   ,  \"τ1\" -> 0.020016820130   ,  \"τS\" -> 0.013372894745   ,  \"τN\" -> 0.000454586591   ,  \"τC\" -> 0.005292751338   ,  \"κ0\" -> 0.000000007771   ,  \"mm1\" -> 0.000078663474   ,  \"mm2\" -> 0.016609276996   ,  \"mm3\" -> 0.022739072051   ,  \"T\" -> 1.100000000000   ,  \"B\" -> 12.000000000000   ,  \"θ\" -> 90.000000000000   ,  \"Reoff\" -> 0.000000000000   ,  \"Imoff\" -> 0.000000000000   ,  \"στ1\" -> 0.000000000000   ,  \"στS\" -> 0.000000000000   ,  \"στN\" -> 0.000000000000    |>   , \r\"IDS0193_210310_RAW_cal__sam_\" ->   <|    \"ζ\" -> 0.014495870556   ,  \"τ1\" -> 0.019990087457   ,  \"τS\" -> 0.016832201384   ,  \"τN\" -> 0.000455517238   ,  \"τC\" -> 0.005555782498   ,  \"κ0\" -> 0.000000008420   ,  \"mm1\" -> 0.000060055560   ,  \"mm2\" -> 0.018114231010   ,  \"mm3\" -> 0.024909902538   ,  \"T\" -> 1.100000000000   ,  \"B\" -> 12.000000000000   ,  \"θ\" -> 90.000000000000   ,  \"Reoff\" -> 0.000000000000   ,  \"Imoff\" -> 0.000000000000   ,  \"στ1\" -> 0.000000000000   ,  \"στS\" -> 0.000000000000   ,  \"στN\" -> 0.000000000000    |>   , \r\"IDS0194_210310_RAW_cal__ref_\" ->   <|    \"ζ\" -> 0.020900896759   ,  \"τ1\" -> 0.018288874472   ,  \"τS\" -> 0.009095511262   ,  \"τN\" -> 0.000107884456   ,  \"τC\" -> 0.006896232004   ,  \"κ0\" -> 0.000000013449   ,  \"mm1\" -> 0.000081424831   ,  \"mm2\" -> 0.015492573296   ,  \"mm3\" -> 0.019006863291   ,  \"T\" -> 1.800000000000   ,  \"B\" -> 12.000000000000   ,  \"θ\" -> 90.000000000000   ,  \"Reoff\" -> 0.000000000000   ,  \"Imoff\" -> 0.000000000000   ,  \"στ1\" -> 0.000000000000   ,  \"στS\" -> 0.000000000000   ,  \"στN\" -> 0.000000000000    |>   , \r\"IDS0194_210310_RAW_cal__sam_\" ->   <|    \"ζ\" -> 0.014043763709   ,  \"τ1\" -> 0.018292068543   ,  \"τS\" -> 0.011311396743   ,  \"τN\" -> 0.000128802259   ,  \"τC\" -> 0.008087849636   ,  \"κ0\" -> 0.000000014258   ,  \"mm1\" -> 0.000065912054   ,  \"mm2\" -> 0.017276417784   ,  \"mm3\" -> 0.020638450794   ,  \"T\" -> 1.800000000000   ,  \"B\" -> 12.000000000000   ,  \"θ\" -> 90.000000000000   ,  \"Reoff\" -> 0.000000000000   ,  \"Imoff\" -> 0.000000000000   ,  \"στ1\" -> 0.000000000000   ,  \"στS\" -> 0.000000000000   ,  \"στN\" -> 0.000000000000    |>   , \r\"IDS0195_210310_RAW_cal__ref_\" ->   <|    \"ζ\" -> 0.019765118173   ,  \"τ1\" -> 0.018324978618   ,  \"τS\" -> 0.006054329354   ,  \"τN\" -> 0.000028420666   ,  \"τC\" -> 0.006398306925   ,  \"κ0\" -> 0.000000023958   ,  \"mm1\" -> 0.000061197185   ,  \"mm2\" -> 0.012449996348   ,  \"mm3\" -> 0.018415068303   ,  \"T\" -> 3.000000000000   ,  \"B\" -> 12.000000000000   ,  \"θ\" -> 90.000000000000   ,  \"Reoff\" -> 0.000000000000   ,  \"Imoff\" -> 0.000000000000   ,  \"στ1\" -> 0.000000000000   ,  \"στS\" -> 0.000000000000   ,  \"στN\" -> 0.000000000000    |>   , \r\"IDS0195_210310_RAW_cal__sam_\" ->   <|    \"ζ\" -> 0.016187684631   ,  \"τ1\" -> 0.018325345271   ,  \"τS\" -> 0.007510087776   ,  \"τN\" -> 0.000028419157   ,  \"τC\" -> 0.008115463080   ,  \"κ0\" -> 0.000000024747   ,  \"mm1\" -> 0.000062903858   ,  \"mm2\" -> 0.015524812312   ,  \"mm3\" -> 0.018513630087   ,  \"T\" -> 3.000000000000   ,  \"B\" -> 12.000000000000   ,  \"θ\" -> 90.000000000000   ,  \"Reoff\" -> 0.000000000000   ,  \"Imoff\" -> 0.000000000000   ,  \"στ1\" -> 0.000000000000   ,  \"στS\" -> 0.000000000000   ,  \"στN\" -> 0.000000000000    |>   , \r\"IDS0196_210310_RAW_cal__ref_\" ->   <|    \"ζ\" -> 0.030164668817   ,  \"τ1\" -> 0.012822215558   ,  \"τS\" -> 0.004108197943   ,  \"τN\" -> 0.000006999504   ,  \"τC\" -> 0.004420975765   ,  \"κ0\" -> 0.000000058872   ,  \"mm1\" -> 0.000063783415   ,  \"mm2\" -> 0.008574867378   ,  \"mm3\" -> 0.012843871546   ,  \"T\" -> 5.700000000000   ,  \"B\" -> 12.000000000000   ,  \"θ\" -> 90.000000000000   ,  \"Reoff\" -> 0.000000000000   ,  \"Imoff\" -> 0.000000000000   ,  \"στ1\" -> 0.000000000000   ,  \"στS\" -> 0.000000000000   ,  \"στN\" -> 0.000000000000    |>   , \r\"IDS0196_210310_RAW_cal__sam_\" ->   <|    \"ζ\" -> 0.027897403691   ,  \"τ1\" -> 0.014639690770   ,  \"τS\" -> 0.004105291179   ,  \"τN\" -> 0.000006999171   ,  \"τC\" -> 0.007414449545   ,  \"κ0\" -> 0.000000059701   ,  \"mm1\" -> 0.000073450671   ,  \"mm2\" -> 0.011534391407   ,  \"mm3\" -> 0.014673310811   ,  \"T\" -> 5.700000000000   ,  \"B\" -> 12.000000000000   ,  \"θ\" -> 90.000000000000   ,  \"Reoff\" -> 0.000000000000   ,  \"Imoff\" -> 0.000000000000   ,  \"στ1\" -> 0.000000000000   ,  \"στS\" -> 0.000000000000   ,  \"στN\" -> 0.000000000000    |>   , \r\"IDS0208_210310_RAW_cal__ref_\" ->   <|    \"ζ\" -> 0.000000000000   ,  \"τ1\" -> 0.000000000000   ,  \"τS\" -> 0.000000000000   ,  \"τN\" -> 0.000000000000   ,  \"τC\" -> 0.000000000000   ,  \"κ0\" -> 0.000000000000   ,  \"mm1\" -> 0.000000000000   ,  \"mm2\" -> 0.000000000000   ,  \"mm3\" -> 0.000000000000   ,  \"T\" -> 0.197000000000   ,  \"B\" -> 0.000000000000   ,  \"θ\" -> 0.000000000000   ,  \"Reoff\" -> 0.000000000000   ,  \"Imoff\" -> 0.000000000000   ,  \"στ1\" -> 0.000000000000   ,  \"στS\" -> 0.000000000000   ,  \"στN\" -> 0.000000000000    |>   , \r\"IDS0208_210310_RAW_cal__sam_\" ->   <|    \"ζ\" -> 0.000000000000   ,  \"τ1\" -> 0.000000000000   ,  \"τS\" -> 0.000000000000   ,  \"τN\" -> 0.000000000000   ,  \"τC\" -> 0.000000000000   ,  \"κ0\" -> 0.000000000000   ,  \"mm1\" -> 0.000000000000   ,  \"mm2\" -> 0.000000000000   ,  \"mm3\" -> 0.000000000000   ,  \"T\" -> 0.197000000000   ,  \"B\" -> 0.000000000000   ,  \"θ\" -> 0.000000000000   ,  \"Reoff\" -> 0.000000000000   ,  \"Imoff\" -> 0.000000000000   ,  \"στ1\" -> 0.000000000000   ,  \"στS\" -> 0.000000000000   ,  \"στN\" -> 0.000000000000    |>   , \r\"IDS0209_210310_RAW_cal__ref_\" ->   <|    \"ζ\" -> 0.163571654798   ,  \"τ1\" -> 0.020520714675   ,  \"τS\" -> 0.073117323271   ,  \"τN\" -> 0.020627224399   ,  \"τC\" -> 0.001336341391   ,  \"κ0\" -> 0.000000001061   ,  \"mm1\" -> 0.000185345173   ,  \"mm2\" -> 0.015331340913   ,  \"mm3\" -> 0.115418868440   ,  \"T\" -> 0.197000000000   ,  \"B\" -> 0.000000000000   ,  \"θ\" -> 0.000000000000   ,  \"Reoff\" -> 0.000000000000   ,  \"Imoff\" -> 0.000000000000   ,  \"στ1\" -> 0.000000000000   ,  \"στS\" -> 0.000000000000   ,  \"στN\" -> 0.000000000000    |>   , \r\"IDS0209_210310_RAW_cal__sam_\" ->   <|    \"ζ\" -> 0.132901556203   ,  \"τ1\" -> 0.022795175616   ,  \"τS\" -> 0.082481385864   ,  \"τN\" -> 0.041432545456   ,  \"τC\" -> 0.001408424074   ,  \"κ0\" -> 0.000000001182   ,  \"mm1\" -> 0.000163042447   ,  \"mm2\" -> 0.014386869823   ,  \"mm3\" -> 0.150035973048   ,  \"T\" -> 0.197000000000   ,  \"B\" -> 0.000000000000   ,  \"θ\" -> 0.000000000000   ,  \"Reoff\" -> 0.000000000000   ,  \"Imoff\" -> 0.000000000000   ,  \"στ1\" -> 0.000000000000   ,  \"στS\" -> 0.000000000000   ,  \"στN\" -> 0.000000000000    |>   , \r\"IDS0210_210310_RAW_cal__ref_\" ->   <|    \"ζ\" -> 0.273010901258   ,  \"τ1\" -> 0.070915437755   ,  \"τS\" -> 0.135576844083   ,  \"τN\" -> 0.040129116812   ,  \"τC\" -> 0.000992387299   ,  \"κ0\" -> 0.000000000644   ,  \"mm1\" -> 0.000211869147   ,  \"mm2\" -> 0.050134062949   ,  \"mm3\" -> 0.245237496593   ,  \"T\" -> 0.148000000000   ,  \"B\" -> 6.000000000000   ,  \"θ\" -> 0.000000000000   ,  \"Reoff\" -> -60040816.326530613000   ,  \"Imoff\" -> 0.000000000000   ,  \"στ1\" -> 0.064590057493   ,  \"στS\" -> 0.016412482982   ,  \"στN\" -> 0.016122106456    |>   , \r\"IDS0210_210310_RAW_cal__sam_\" ->   <|    \"ζ\" -> 0.000000000000   ,  \"τ1\" -> 0.000000000000   ,  \"τS\" -> 0.000000000000   ,  \"τN\" -> 0.000000000000   ,  \"τC\" -> 0.000000000000   ,  \"κ0\" -> 0.000000000000   ,  \"mm1\" -> 0.000000000000   ,  \"mm2\" -> 0.000000000000   ,  \"mm3\" -> 0.000000000000   ,  \"T\" -> 0.148000000000   ,  \"B\" -> 6.000000000000   ,  \"θ\" -> 0.000000000000   ,  \"Reoff\" -> 0.000000000000   ,  \"Imoff\" -> 0.000000000000   ,  \"στ1\" -> 0.000000000000   ,  \"στS\" -> 0.000000000000   ,  \"στN\" -> 0.000000000000    |>   , \r\"IDS0211_210310_RAW_cal__ref_\" ->   <|    \"ζ\" -> 0.160882265826   ,  \"τ1\" -> 0.034919932965   ,  \"τS\" -> 0.043973777096   ,  \"τN\" -> 0.047289018614   ,  \"τC\" -> 0.001339652100   ,  \"κ0\" -> 0.000000001069   ,  \"mm1\" -> 0.000181515969   ,  \"mm2\" -> 0.014272071349   ,  \"mm3\" -> 0.127751358817   ,  \"T\" -> 0.197000000000   ,  \"B\" -> 9.000000000000   ,  \"θ\" -> 0.000000000000   ,  \"Reoff\" -> 0.000000000000   ,  \"Imoff\" -> 0.000000000000   ,  \"στ1\" -> 0.000000000000   ,  \"στS\" -> 0.000000000000   ,  \"στN\" -> 0.000000000000    |>   , \r\"IDS0211_210310_RAW_cal__sam_\" ->   <|    \"ζ\" -> 0.132534999612   ,  \"τ1\" -> 0.042581417401   ,  \"τS\" -> 0.054103824371   ,  \"τN\" -> 0.072163013930   ,  \"τC\" -> 0.001421040158   ,  \"κ0\" -> 0.000000001190   ,  \"mm1\" -> 0.000162934689   ,  \"mm2\" -> 0.015546305497   ,  \"mm3\" -> 0.171294831040   ,  \"T\" -> 0.197000000000   ,  \"B\" -> 9.000000000000   ,  \"θ\" -> 0.000000000000   ,  \"Reoff\" -> 0.000000000000   ,  \"Imoff\" -> 0.000000000000   ,  \"στ1\" -> 0.000000000000   ,  \"στS\" -> 0.000000000000   ,  \"στN\" -> 0.000000000000    |>   , \r\"IDS0212_210310_RAW_cal__ref_\" ->   <|    \"ζ\" -> 0.154351103049   ,  \"τ1\" -> 0.051844552801   ,  \"τS\" -> 0.034651211615   ,  \"τN\" -> 0.065884588100   ,  \"τC\" -> 0.001166375427   ,  \"κ0\" -> 0.000000001084   ,  \"mm1\" -> 0.000152080810   ,  \"mm2\" -> 0.013701664106   ,  \"mm3\" -> 0.155210794609   ,  \"T\" -> 0.197000000000   ,  \"B\" -> 11.000000000000   ,  \"θ\" -> 0.000000000000   ,  \"Reoff\" -> 0.000000000000   ,  \"Imoff\" -> 0.000000000000   ,  \"στ1\" -> 0.000000000000   ,  \"στS\" -> 0.000000000000   ,  \"στN\" -> 0.000000000000    |>   , \r\"IDS0212_210310_RAW_cal__sam_\" ->   <|    \"ζ\" -> 0.124414912597   ,  \"τ1\" -> 0.052685716706   ,  \"τS\" -> 0.041788480794   ,  \"τN\" -> 0.092820346766   ,  \"τC\" -> 0.001183564004   ,  \"κ0\" -> 0.000000001217   ,  \"mm1\" -> 0.000128067207   ,  \"mm2\" -> 0.013191279693   ,  \"mm3\" -> 0.191906106886   ,  \"T\" -> 0.197000000000   ,  \"B\" -> 11.000000000000   ,  \"θ\" -> 0.000000000000   ,  \"Reoff\" -> 0.000000000000   ,  \"Imoff\" -> 0.000000000000   ,  \"στ1\" -> 
